vi "Send Command.vi"(8 "error in (no error)":errorcluster, 10 "write buffer":string, 11 "VISA resource name":refnum<visa-resource-name>) -> (0 "error out":errorcluster, 3 "VISA resource name out":refnum<visa-resource-name>)   [LabVIEW 2017, in "Agilent PSG MXG Series.lvlib"]
uses:
  Agilent PSG MXG Series.lvlib
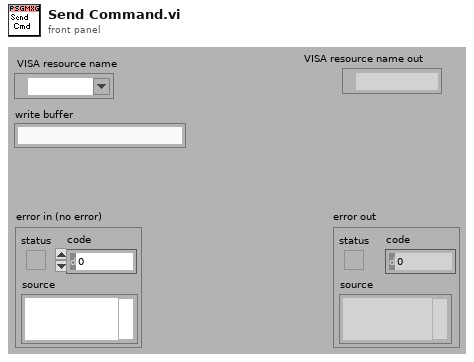
[diagram p1: front panel]
types:
  T1 = typedef "Semaphore RefNum" = refnum<k1>
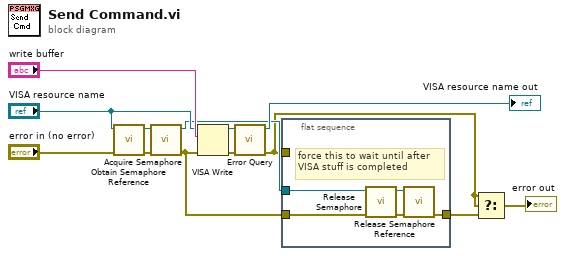
[diagram p0: block diagram]
diagram:
  n1 = call <vilib>:"Obtain Semaphore Reference.vi"("error in (no error)"="error in (no error)", "name (unnamed)"="VISA resource name") -> ("error out"=w10:errorcluster, "semaphore"=w11:T1)  [unwired: 1 in, 3 out]
  n2 = call <vilib>:"Acquire Semaphore.vi"("error in (no error)"=w10, "semaphore"=w11) -> ("error out"=w3:errorcluster, "semaphore out"=w8:T1)  [unwired: 1 in, 3 out]
  n3 = VISA Write(VISA resource name="VISA resource name", write buffer="write buffer", error in (no error)=w3) -> (VISA resource name out=w5:refnum<visa-resource-name>, error out=w6:errorcluster)  [unwired: 1 out]
  n4 = call "Error Query.vi"("error in (no error)"=w6, "VISA resource name"=w5) -> ("error out"=w4:errorcluster, "VISA resource name out"=→"VISA resource name out":refnum<visa-resource-name>)  [unwired: 8 out]
  n5 = flat-sequence {
    tunnel: w8 -> [w18]
    tunnel: [w15] -> w2
    tunnel: w4 -> [_]
    tunnel: w3 -> [w14]
    frame #0 {
      # "force this to wait until after \nVISA stuff is completed"
      n6 = call <vilib>:"Release Semaphore.vi"("error in (no error)"=w14, "semaphore"=w18) -> ("error out"=w16:errorcluster, "semaphore out"=w17:T1)  [unwired: 4 out]
      n7 = call <vilib>:"Release Semaphore Reference.vi"("error in (no error)"=w16, "semaphore"=w17) -> ("error out"=w15:errorcluster)  [unwired: 9 out]
    }
  }
  n8 = Select(t=w4, s=w4, f=w2) -> (s? t:f=→"error out":errorcluster)
